vi "Initialize Class.vi"(8 "error in (no error)":errorcluster, 11 "DataQueues in":refnum<class "DataQueues.lvclass">) -> (0 "error out":errorcluster, 3 "DataQueues out":refnum<class "DataQueues.lvclass">)   [LabVIEW 2017, in "DataQueues.lvclass"]
doc: "Developed by Kevin Thompson\nkevin@thompsonengineering.net\n\nCopyright 2018-2020\nThompson Engineering, LLC"
uses:
  DataQueues.lvclass
  DataTypes/Object Data--cluster.ctl
  DataQueues.lvclass/DataQueues.ctl
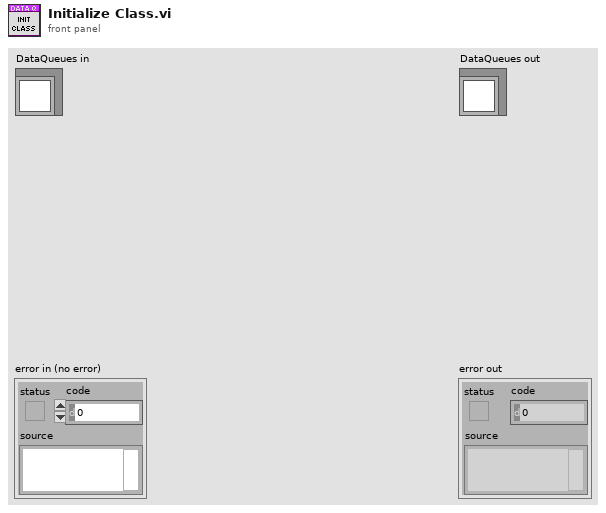
[diagram p1: front panel]
types:
  T1 = typedef "DataQueues.lvclass/Object Data--cluster.ctl" = cluster{"QueueNames":string[]}
  T2 = typedef "TD Dynamic CVT DVR--ref.ctl" = refnum<data-value>
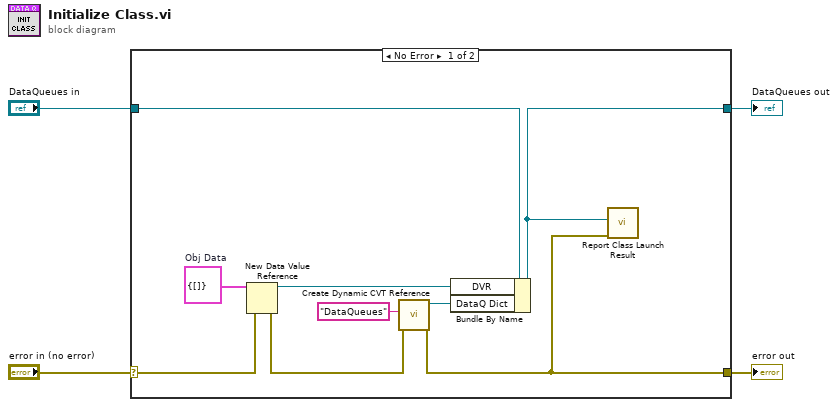
[diagram p0: block diagram]
diagram:
  n1 = case shown="No Error" "error in (no error)" {
    selector: "error in (no error)" -> [w10 w15]
    tunnel: [w5 w15] -> w3
    tunnel: [w6 w14] -> w1
    tunnel: "DataQueues in" -> [w7 w14]
    frame No Error {
      w11 = T1 {"QueueNames"=[]}  # Obj Data
      n2 = New Data Value Reference(data value=w11, error in=w10) -> (data value reference=w8:refnum<data-value>, error out=w9:errorcluster)
      n3 = call <vilib>:"Create Dynamic CVT Reference.vi"("error in (no error)"=w9, "DictName"="DataQueues") -> ("error out"=w5:errorcluster, "dCVT DVR out"=w12:T2)  [unwired: 8 in]
      n4 = Bundle By Name(cluster=w7, "DVR"=w8, "DataQ Dict"=w12) -> (w6:refnum<class "DataQueues.lvclass">)
      n5 = call "Report Class Launch Result.vi"("Object"=w6, "error in (no error)"=w5) -> ()  [unwired: 8 in, 1 out]
    }
    frame Error {
    }
  }
  "error out" <- w3
  "DataQueues out" <- w1
